vi "POSITION ARM STROKE.vi"(0 "PhoenixMotorControlDevRef":T2={"DeviceStatus"={"status"=FALSE, "code"=0, "source"=""}, "Type"=enum."PWM", "PWM"={"PWM Channel"=enum."PWM 1", "DeadBand"={"Name"="", "maxPositivePwm"=0, "minPositivePwm"=0, "centerPwm"=0, "maxNegativePwm"=0, "minNegativePwm"=0, "angularRange"=0}}, "CAN"={"Device Number"=0, "SetOutput VI Ref"=variant(enum8{"Percent VBus", "Current", "Speed", "Position", "Voltage"} enum."Percent VBus"), "GetOutput VI Ref"=variant(refnum<k1> refnum), "Enable VI Ref"=variant(dbl 12.0), "Disable VI Ref"=variant(enum8{"Percent VBus", "Speed", "Position", "Slave", "Unchanged / Invalid", "Voltage Compensation", "Current", "Motion Profile"} enum."Percent VBus"), "Data"=variant}, "Invert"=FALSE, "DIO PWM"={"PWM \"Enable\" Channel"=enum."Invalid", "DIOChannel"=enum."Invalid", "PWM Rate"=0.0}}, 1 "arm angle table":T1, 5 "target position (tics)":dbl=40960.0 format="%#_13g", 9 "arm angle motor pos":dbl, 11 "error in (no error)":errorcluster, 12 "PID Constants":T7={"P Gain"=0.5, "I Gain"=0.0, "D Gain"=0.0, "F Gain"=0.0, "I Zone"=0.0, "Min Output"=-1.0, "Max Output"=1.0} {"Max Output" min=-1.0 max=1.0 step=0.01; "Min Output" min=-1.0 max=1.0 step=0.01; "I Zone" step=0.01; "F Gain" step=0.01; "D Gain" step=0.01; "I Gain" step=0.01; "P Gain" min=0.0 step=0.01}, 13 "tics per inch":dbl=18774.68103 format="%#_13g", 14 "Falcon 500 tics per rev":dbl=2048.0 format="%#_13g") -> (4 "PhoenixMotorControlDevRef 2":T2={"DeviceStatus"={"status"=FALSE, "code"=0, "source"=""}, "Type"=enum."PWM", "PWM"={"PWM Channel"=enum."PWM 1", "DeadBand"={"Name"="", "maxPositivePwm"=0, "minPositivePwm"=0, "centerPwm"=0, "maxNegativePwm"=0, "minNegativePwm"=0, "angularRange"=0}}, "CAN"={"Device Number"=0, "SetOutput VI Ref"=variant(enum8{"Percent VBus", "Current", "Speed", "Position", "Voltage"} enum."Percent VBus"), "GetOutput VI Ref"=variant(refnum<k1> refnum), "Enable VI Ref"=variant(dbl 12.0), "Disable VI Ref"=variant(enum8{"Percent VBus", "Speed", "Position", "Slave", "Unchanged / Invalid", "Voltage Compensation", "Current", "Motion Profile"} enum."Percent VBus"), "Data"=variant}, "Invert"=FALSE, "DIO PWM"={"PWM \"Enable\" Channel"=enum."Invalid", "DIOChannel"=enum."Invalid", "PWM Rate"=0.0}}, 15 "error out":errorcluster)   [LabVIEW 2020]
uses:
  <vilib>/Rock Robotics/WPI/MotorControl/WPI_MotorControlDeviceRef.ctl
  <vilib>/Rock Robotics/WPI/MotorControl/WPI_MotorControlType.ctl
  <vilib>/Rock Robotics/SystemInterfaces/DIO/FPGA_DIOPWMChannel.ctl
  <vilib>/Rock Robotics/WPI/PWM/WPI_PWMDeadband.ctl
  <vilib>/Rock Robotics/SystemInterfaces/DIO/FPGA_DIOChannel.ctl
  <vilib>/Rock Robotics/WPI/ThirdParty/Phoenix-LabVIEW/Motor Controller/Controls/CTRE_Phoenix_MotorControl_ControlMode.ctl
  <vilib>/Rock Robotics/WPI/ThirdParty/Phoenix-LabVIEW/Motor Controller/Get/CTRE_Phoenix_MotorController_GetVoltage.vi
  <vilib>/Rock Robotics/WPI/ThirdParty/Phoenix-LabVIEW/Motor Controller/Get/CTRE_Phoenix_MotorController_IntegratedSensorData_TalonFX.vi
  <vilib>/Analysis/NI_AALPro.lvlib
panel:
  out "MAX stroke length":dbl format="%0.2f"
  out "SensorPos (tics)":i32
  out "Target Position (tics)":dbl
  out "Sensor Velocity (rpm)":i32
  out "Applied Output":dbl
  out "Position Closed Loop Plots":cluster{dbl, "Position":dbl}(graph)
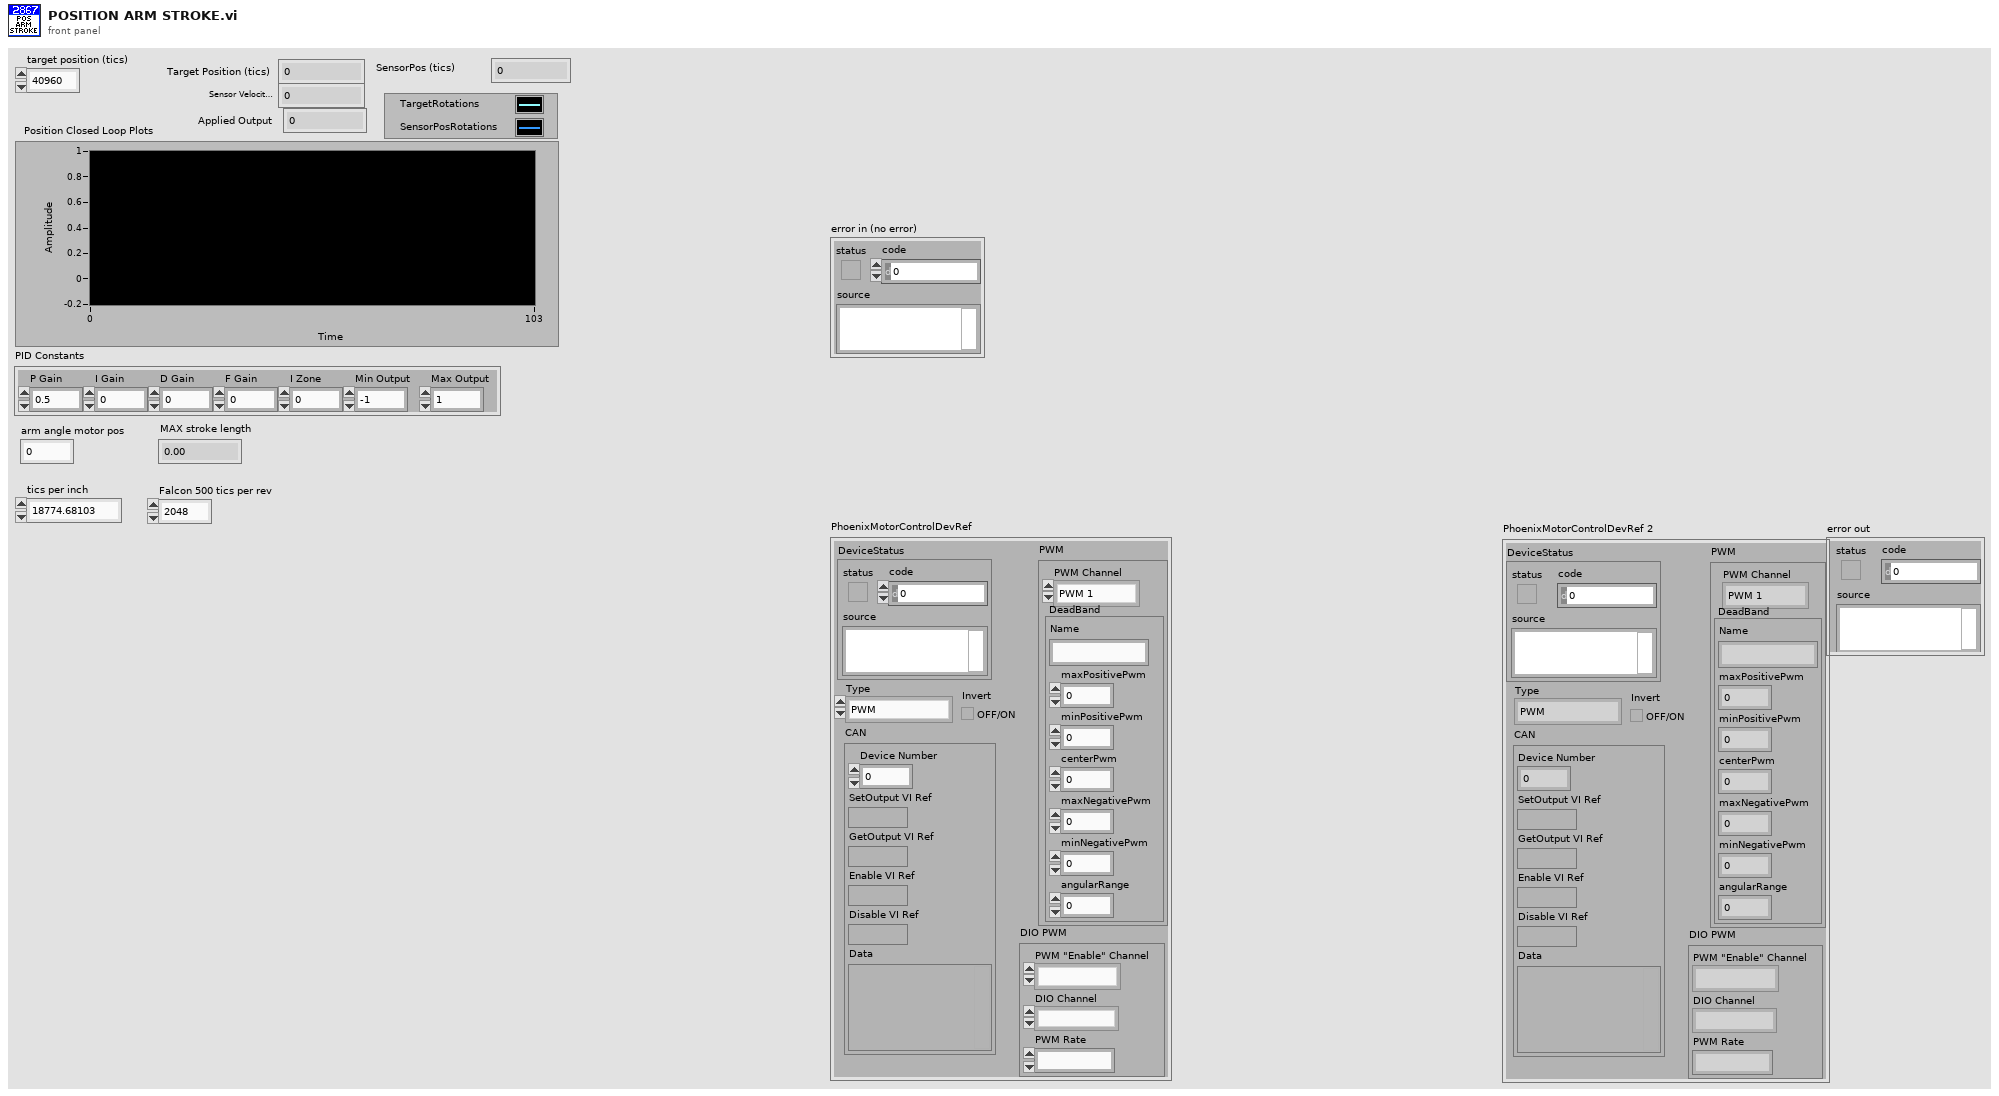
[diagram p1: front panel]
types:
  T1 = cluster{"X pos (in)":dbl[], "arm angle (deg)":dbl[], "ht LIMIT (in)":dbl[], "ht HANGAR (in)":dbl[]}
  T2 = typedef "WPI_MotorControlDeviceRef.ctl" = cluster{"DeviceStatus":errorcluster, "Type":T3, "PWM":cluster{"PWM Channel":T4, "DeadBand":T5}, "CAN":cluster{"Device Number":u8, "SetOutput VI Ref":variant, "GetOutput VI Ref":variant, "Enable VI Ref":variant, "Disable VI Ref":variant, "Data":variant}, "Invert":bool, "DIO PWM":cluster{"PWM \"Enable\" Channel":T4, "DIOChannel":T6, "PWM Rate":dbl}}
  T3 = typedef "WPI_MotorControlType.ctl" = enum16{"PWM", "CAN", "DIO PWM"}
  T4 = typedef "FPGA_DIOPWMChannel.ctl" = enum8{"PWM 0", "PWM 1", "PWM 2", "PWM 3", "PWM 4", "PWM 5", "PWM 6", "PWM 7", "PWM 8", "PWM 9", "PWM MXP 0", "PWM MXP 1", "PWM MXP 2", "PWM MXP 3", "PWM MXP 4", "PWM MXP 5", "PWM MXP 6", "PWM MXP 7", "PWM MXP 8", "PWM MXP 9", "Invalid"}
  T5 = typedef "WPI_PWMDeadband.ctl" = cluster{"Name":string, "maxPositivePwm":i32, "minPositivePwm":i32, "centerPwm":i32, "maxNegativePwm":i32, "minNegativePwm":i32, "angularRange":u16}
  T6 = typedef "FPGA_DIOChannel.ctl" = enum8{"DIO 0", "DIO 1", "DIO 2", "DIO 3", "DIO 4", "DIO 5", "DIO 6", "DIO 7", "DIO 8", "DIO 9", "DIO MXP 0", "DIO MXP 1", "DIO MXP 2", "DIO MXP 3", "DIO MXP 4", "DIO MXP 5", "DIO MXP 6", "DIO MXP 7", "DIO MXP 8", "DIO MXP 9", "DIO MXP 10", "DIO MXP 11", "DIO MXP 12", "DIO MXP 13", "DIO MXP 14", "DIO MXP 15", "SPI Port CS1", "SPI Port CS2", "SPI Port CS3", "SPI Port MISO", "SPI Port MOSI", "Invalid"}
  T7 = cluster{"P Gain":dbl, "I Gain":dbl, "D Gain":dbl, "F Gain":dbl, "I Zone":dbl, "Min Output":dbl, "Max Output":dbl}
  T8 = typedef "CTRE_Phoenix_MotorControl_ControlMode.ctl" = u16
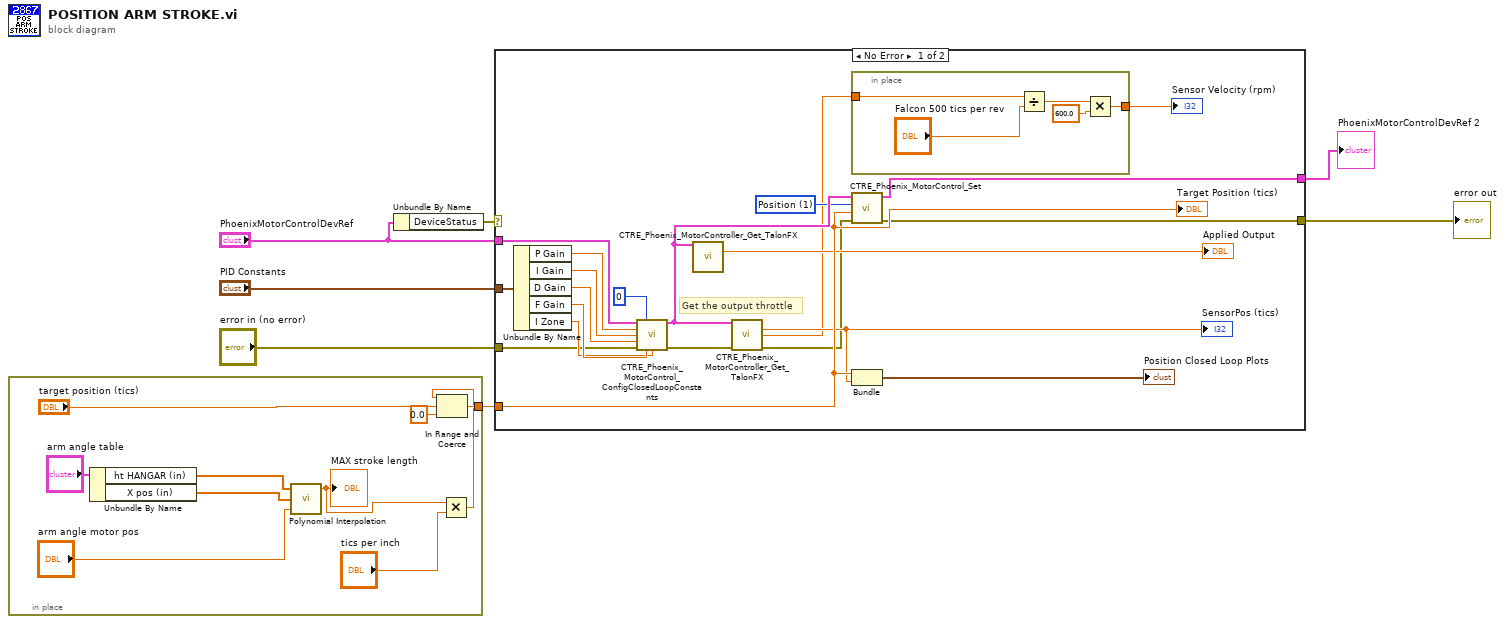
[diagram p0: block diagram]
diagram:
  n1 = in-place {
    in-place-border: [w10] -> w1
    n2 = Unbundle By Name("arm angle table") -> ("ht HANGAR (in)"=w15:dbl[], "X pos (in)"=w14:dbl[])
    n3 = call <vilib>:"Polynomial Interpolation.vi"("x value"="arm angle motor pos", "X"=w14, "Y"=w15) -> ("interpolation value"=w12:dbl)  [unwired: 2 out]
    "MAX stroke length" <- w12
    n4 = Multiply(x=w12, y="tics per inch") -> (x*y=w8:dbl)
    n5 = In Range and Coerce(upper limit=w8, x="target position (tics)", lower limit=0.0) -> (coerced(x)=w10:dbl)  [unwired: 1 out]
  }
  n6 = Unbundle By Name("PhoenixMotorControlDevRef") -> ("DeviceStatus"=w5:errorcluster)
  n7 = case shown="No Error" w5 {
    tunnel: w1 -> [w37 _]
    tunnel: "PhoenixMotorControlDevRef" -> [w31 _]
    tunnel: "PID Constants" -> [w29 _]
    tunnel: [w22 _] -> w4
    tunnel: [w21 _] -> w3
    tunnel: "error in (no error)" -> [w18 _]
    frame No Error {
      w32 = T8 1 items=["PercentOutput"=0, "Position"=1, "Velocity"=2, "Follower"=5, "MotionProfile"=6, "MotionMagic"=7, "MotionMagicArc"=8, "TimedPercentOutput"=9, "Disabled"=15] ("Control Mode")
      # "Get the output throttle"
      n8 = Unbundle By Name(w29) -> ("P Gain"=w28:dbl, "I Gain"=w27:dbl, "D Gain"=w26:dbl, "F Gain"=w25:dbl, "I Zone"=w24:dbl)
      n9 = call <vilib>:"CTRE_Phoenix_MotorControl_ConfigClosedLoopConstants.vi"("PhoenixMotorControlDevRef"=w31, "slotIdx"=0, "P"=w28, "I"=w27, "D"=w26, "error in (no error)"=w18, "F"=w25, "I Zone"=w24) -> ("PhoenixMotorControlDevRef"=w35:T2, "error out"=w20:errorcluster)  [unwired: 6 in]
      n10 = call-poly <vilib>:"CTRE_Phoenix_MotorController_Get_TalonFX.vi"("PhoenixMotorControlDevRef"=w35) -> ("Percent Output"=→"Applied Output":dbl)  [unwired: 10 in, 4 out]
      n11 = call-poly <vilib>:"CTRE_Phoenix_MotorController_Get_TalonFX.vi"("PhoenixMotorControlDevRef"=w35, "error in"=w20) -> ("Position"=w36:dbl, "Velocity"=w30:dbl, "error out"=w19:errorcluster)  [unwired: 9 in, 2 out]
      "SensorPos (tics)" <- w36
      n12 = in-place {
        in-place-border: w30 -> [w43]
        in-place-border: [w40] -> w23
        n13 = Divide(x=w43, y="Falcon 500 tics per rev") -> (x/y=w42:dbl)
        n14 = Multiply(x=w42, y=600.0) -> (x*y=w40:dbl)
      }
      "Sensor Velocity (rpm)" <- w23
      n15 = call <vilib>:"CTRE_Phoenix_MotorControl_Set.vi"("error in (no error)"=w19, "Output"=w37, "Control Mode"=w32, "PhoenixMotorControlDevRef"=w35) -> ("error out"=w22:errorcluster, "PhoenixMotorControlDevRef"=w21:T2)  [unwired: 6 in]
      n16 = Bundle("lower limit"=w37, "Position"=w36) -> (→"Position Closed Loop Plots":cluster{"lower limit":dbl, "Position":dbl})  [unwired: 1 in]
      "Target Position (tics)" <- w37
    }
    frame Error {
    }
  }
  "error out" <- w4
  "PhoenixMotorControlDevRef 2" <- w3
